vi "ISV Calibration.vi"(7 "queue out":refnum<queue>) -> (1 "Channel Values":dbl[](array[numeric]), 2 "Suceeded":bool, 3 "ADC Table":T1[](array[typedef]))   [LabVIEW 2015]
uses:
  Type/_RT Configuration 2.ctl
  Type/_RT Command.ctl
  Print.ctl
  Configuration/_Global Configuration.vi
  <vilib>/printing/EasyPrintingControls.llb/orientation.ctl
  <vilib>/Utility/NIReport.llb/NI_ReportGenerationCore.lvlib
  <vilib>/printing/EasyPrintingControls.llb/panel_scaling_for_page.ctl
  <vilib>/printing/EasyPrintingControls.llb/margin_values.ctl
  <vilib>/printing/EasyPrintingControls.llb/measurement_system.ctl
  <vilib>/printing/EasyPrintingControls.llb/margins.ctl
  <vilib>/printing/EasyPrintingControls.llb/printing_method.ctl
  <vilib>/printing/EasyPrintingControls.llb/color_or_monochrome.ctl
  <vilib>/printing/EasyPrintingControls.llb/printer_options.ctl
  <vilib>/printing/EasyPrintingControls.llb/page_headers.ctl
  <vilib>/printing/EasyPrintingControls.llb/page_header_content_options.ctl
  <vilib>/printing/EasyPrintingControls.llb/page_header_options.ctl
  <vilib>/printing/EasyPrintingControls.llb/layout_options.ctl
  <vilib>/printing/EasyPrinting.llb/Easy Print VI Panel or Documentation (path).vi
panel:
  out "Progress Bar":u8(slide) scale=0.0..8.0
  out "Error Out":errorcluster
  in  "Error In":errorcluster
  in  "Print":bool
  in  "ADC Channel Calibration":string[][](table)=[["CAP", "104", "0", "", "1000"], ["ISV1", "107", "0", "", "5850"], ["ISV2", "109", "0", "", "5850"]]
  in  "Done":bool
  in  "Start":bool
  out "Current Task":string="Press Start Calibration button to begin or Done button to exit"
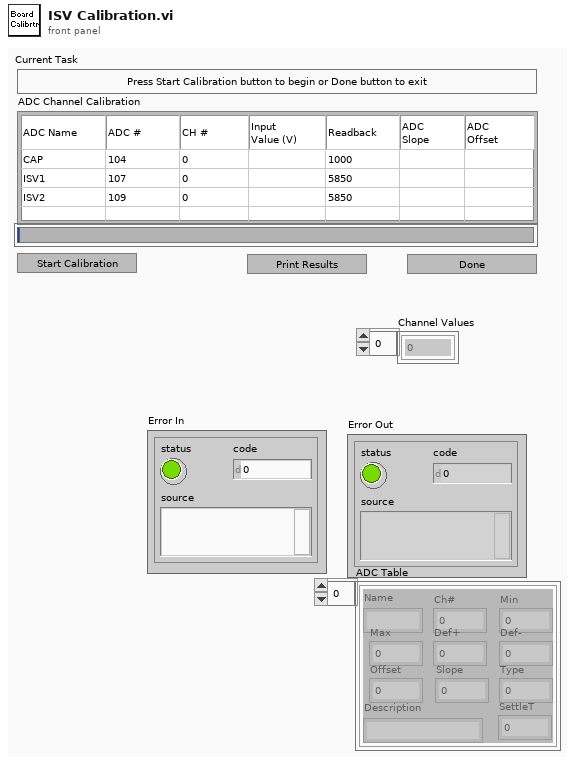
[diagram p1: front panel]
types:
  T1 = typedef "_RT Configuration 2.ctl" = cluster{"Name":string, "Ch#":u8, "Min":dbl, "Max":dbl, "Def+":dbl, "Def-":dbl, "Offset":dbl, "Slope":dbl, "Type":u8, "Description":string, "SettleT":dbl}
  T2 = typedef "_RT Command.ctl" = enum16{"xml Start Run", "xml Start Actual Run", "xml Stop Run", "xml Runtime Update", "xml Get Status", "xml Get Table", "xml Set Table", "xml Get Configuration", "xml System Status", "xml Set LC Input Logic", "xml Get Data", "xml Get Info", "Start", "StartActualRun", "Stop", "Runtime Update", "Get Data", "Get Info", "Get Status", "Get Param", "Get Config", "Get Table", "Read ADC", "Set Oscillator", "Update Config", "Update Table", "Set All Pol", "Set Pol and DC", "Set Max Mass", "Toggle RP", "Toggle EL", "Set PIC", "Initialize Turbo", "Send Turbo Comm", "Close Turbo", "P1", "P2", "P3", "Send Serial", "Set LC Out", "Get LC In", "Read VAC", "Test Table", "Toggle Power", "Get Startup", "Set Startup", "Get ADC Table", "Set ADC Table", "Get Brief Status", "Get Detail Status", "Auxiliary Update", "Set CC Logics", "Set CC Input Logics", "Ignore Error", "invalid"}
  T3 = typedef "Print.ctl" = cluster{"Picture Name":string, "VI Reference":refnum<vi>}
  T4 = typedef "NI_ReportGenerationCore.lvlib/layout_options.ctl" = cluster{"orientation (unchanged)":T5, "panel scaling for page (unchanged)":T6, "margins":T7, "printer options":T10, "page header options":T13}
  T5 = typedef "NI_ReportGenerationCore.lvlib/orientation.ctl" = u16
  T6 = typedef "NI_ReportGenerationCore.lvlib/panel_scaling_for_page.ctl" = u16
  T7 = typedef "NI_ReportGenerationCore.lvlib/margins.ctl" = cluster{"override VI margins (false)":bool, "margins (1.00)":T8, "measurement system (default)":T9}
  T8 = typedef "NI_ReportGenerationCore.lvlib/margin_values.ctl" = cluster{"top":dbl, "left":dbl, "right":dbl, "bottom":dbl}
  T9 = typedef "NI_ReportGenerationCore.lvlib/measurement_system.ctl" = u16
  T10 = typedef "NI_ReportGenerationCore.lvlib/printer_options.ctl" = cluster{"destination printer name (current)":string, "printing method (unchanged)":T11, "color or monochrome (unchanged)":T12}
  T11 = typedef "NI_ReportGenerationCore.lvlib/printing_method.ctl" = u16
  T12 = typedef "NI_ReportGenerationCore.lvlib/color_or_monochrome.ctl" = u16
  T13 = typedef "NI_ReportGenerationCore.lvlib/page_header_options.ctl" = cluster{"page headers (unchanged)":T14, "page header content options":T15}
  T14 = typedef "NI_ReportGenerationCore.lvlib/page_headers.ctl" = u16
  T15 = typedef "NI_ReportGenerationCore.lvlib/page_header_content_options.ctl" = cluster{"Include VI Name":bool, "Include VI Path":bool, "Include Last Modification Date":bool, "Include Date Printed":bool, "Include Page Number":bool, "Include VI Icon":bool}
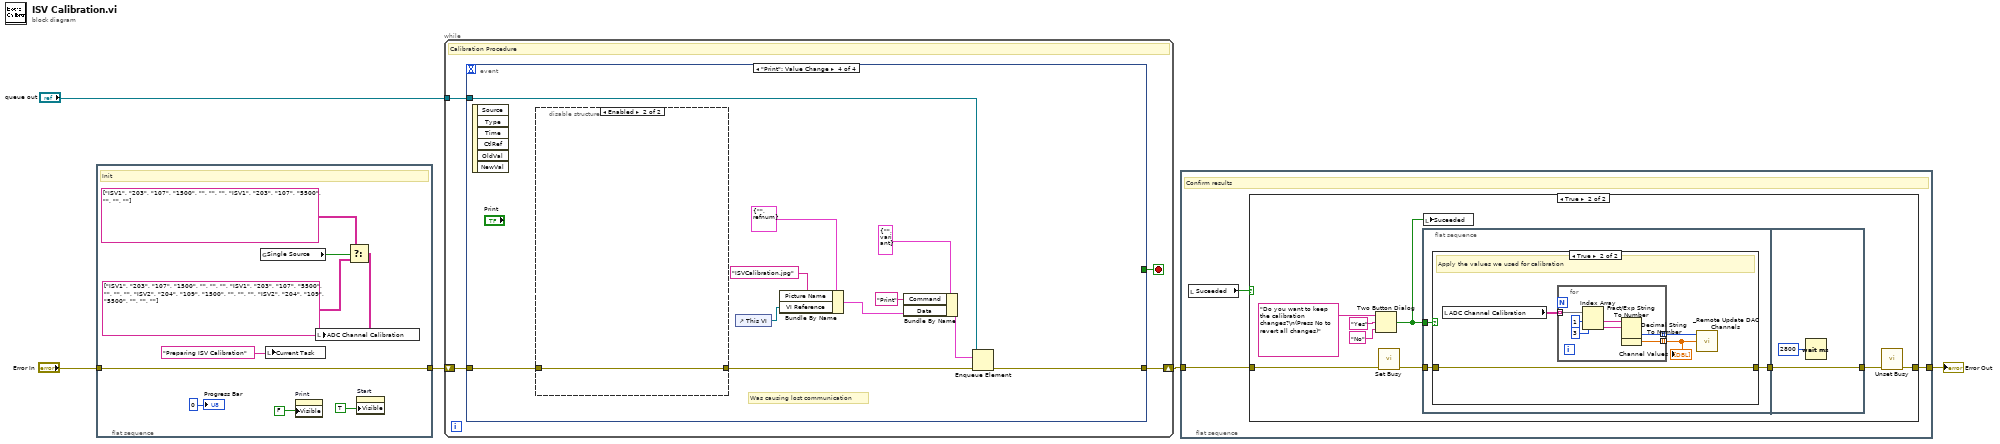
[diagram p0: block diagram]
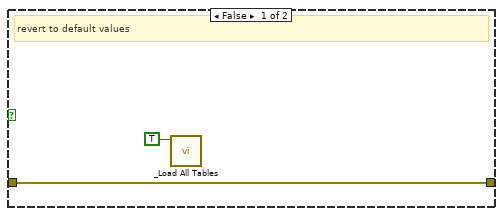
[diagram p3: hidden frame]
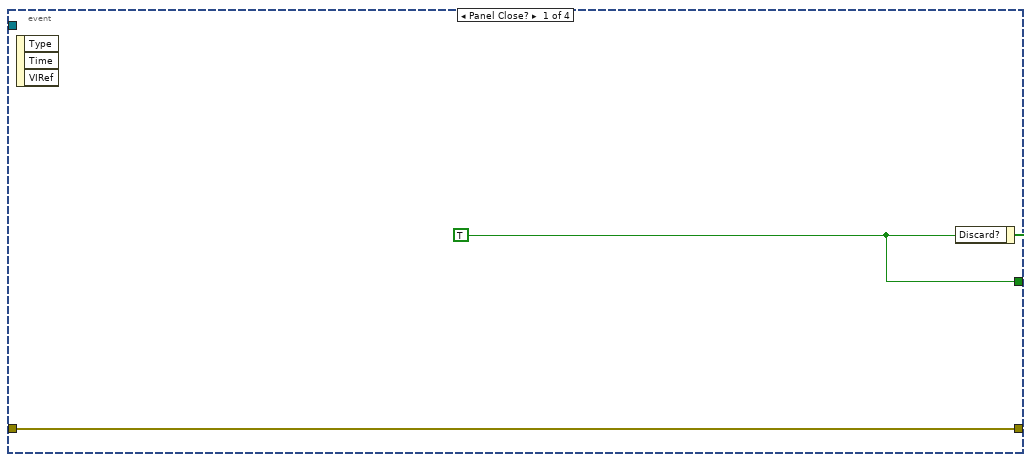
[diagram p4: hidden frame]
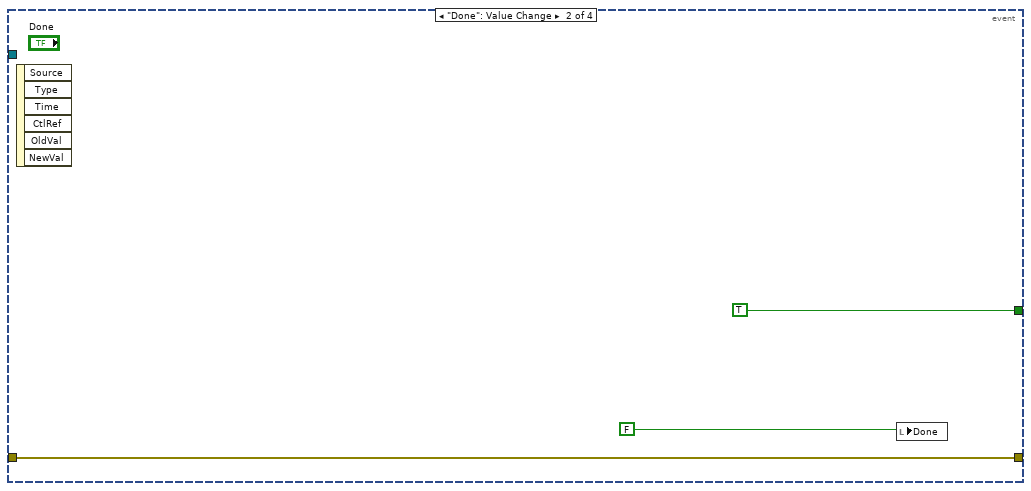
[diagram p5: hidden frame]
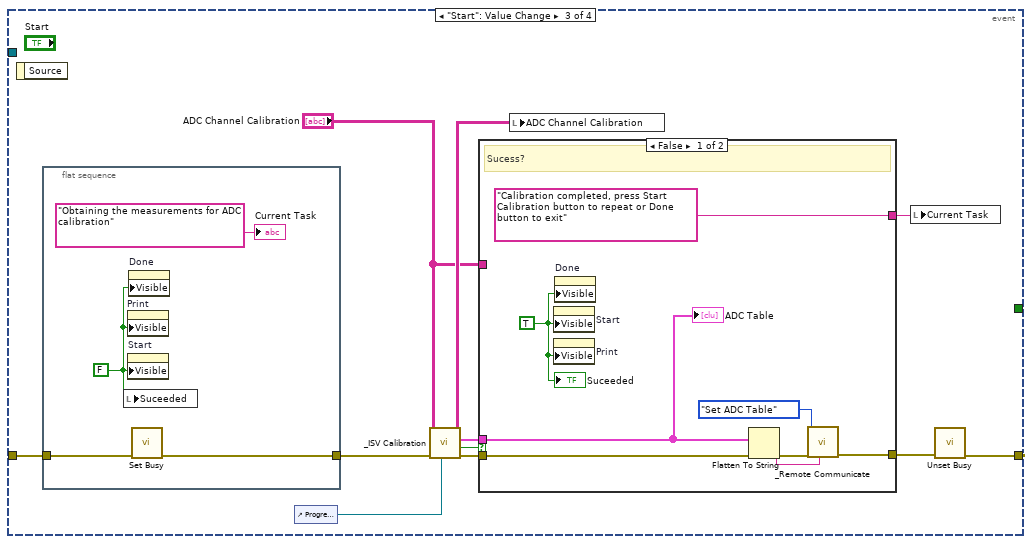
[diagram p6: hidden frame]
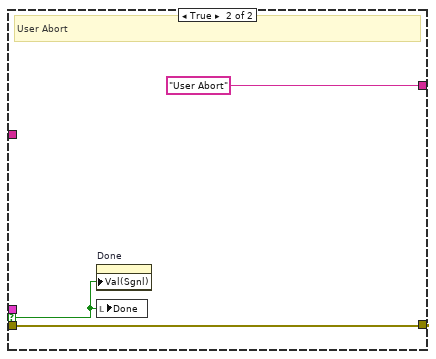
[diagram p7: hidden frame]
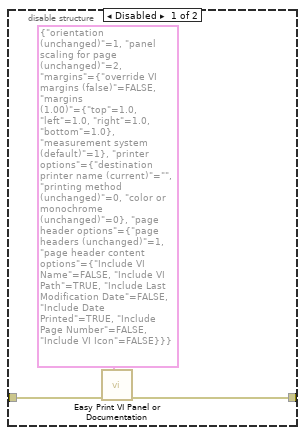
[diagram p8: hidden frame]
diagram:
  n1 = flat-sequence {
    tunnel: "Error In" -> [w11]
    tunnel: [w11] -> w4
    frame #0 {
      # "Init"
      n2 = global read "_Global Configuration.vi" "Single Source"() -> (w10:bool)
      n3 = local write "Current Task"("Preparing ISV Calibration" ("format string")) -> ()
      n4 = property on="Print" class="Bool"("Visible"=FALSE) -> ()  [unwired: 2 in, 2 out]
      n5 = Select(t=string[][] [["ISV1", "203", "107", "1500", "", "", ""], ["ISV1", "203", "107", "5500", "", "", ""]] ("ADC Channel Calibration 2"), s=w10, f=string[][] [["ISV1", "203", "107", "1500", "", "", ""], ["ISV1", "203", "107", "5500", "", "", ""], ["ISV2", "204", "109", "1500", "", "", ""], ["ISV2", "204", "109", "5500", "", "", ""]] ("ADC Channel Calibration 2")) -> (s? t:f=w7:string[][])
      n6 = local write "ADC Channel Calibration"(w7) -> ()
      n7 = property on="Start" class="Bool"("Visible"=TRUE) -> ()  [unwired: 2 in, 2 out]
      "Progress Bar" <- u8 0 ("Progress Bar")
    }
  }
  n8 = while {
    shift-right: [w16] -> w3
    shift-left: w4 -> [w17]
    tunnel: "queue out" -> [w15]
    stop <- w18 stop-if-true
    # "Calibration Procedure"
    n9 = event shown="[3] \"Print\": Value Change" {
      selector: _ -> [_ _ _ _]
      dyn-events: _ -> [_ _ _ _]
      timeout: _ -> [_ _ _ _]
      tunnel: [w20 TRUE _ _] -> w18
      tunnel: w17 -> [w19 w21 w34 w60]
      tunnel: [w19 w21 w33 w58] -> w16
      tunnel: w15 -> [_ _ _ w57]
      event Panel Close? {
        w20 = TRUE
        n10 = event-data() -> ()  [unwired: 4 out]
        n11 = event-data("Discard?"=w20) -> ()  [unwired: 1 in, 1 out]
      }
      event "Done": Value Change {
        n12 = event-data() -> ()  [unwired: 7 out]
        n13 = local write "Done"(FALSE ("Done")) -> ()
      }
      event "Start": Value Change {
        n14 = event-data() -> ()  [unwired: 2 out]
        n15 = flat-sequence {
          tunnel: w34 -> [w38]
          tunnel: [w37] -> w32
          frame #0 {
            w35 = FALSE ("Visible")
            n16 = local write "Suceeded"(w35) -> ()
            n17 = property on="Print" class="Bool"("Visible"=w35) -> ()  [unwired: 2 in, 2 out]
            n18 = property on="Start" class="Bool"("Visible"=w35) -> ()  [unwired: 2 in, 2 out]
            n19 = property on="Done" class="Bool (strict)"("Visible"=w35) -> ()  [unwired: 2 in, 2 out]
            n20 = call <vilib>:"Set Busy.vi"("error in (no error)"=w38) -> ("error out"=w37:errorcluster)  [unwired: 3 in, 7 out]
            "Current Task" <- "Obtaining the measurements for ADC calibration" ("Current Task")
          }
        }
        n21 = control-ref of="Progress Bar"() -> (w24:refnum<vi>)
        n22 = call "_ISV Calibration.vi"("Progress Bar"=w24, "Error In"=w32, "ADC Channel Calibration In"="ADC Channel Calibration") -> ("Error Out"=w31:errorcluster, "aborted"=w30:bool, "ADC Table"=w29:T1[], "ADC Channel Calibration Out"=w26:string[][])  [unwired: 5 in]
        n23 = case shown="False" w30 {
          selector: w30 -> [_ w49]
          tunnel: w31 -> [w45 w48]
          tunnel: w29 -> [w40 _]
          tunnel: [w42 w48] -> w28
          tunnel: ["Calibration completed, press Start Calibration button to repeat or Done button to exit" ("Current Task") "User Abort" ("Current Task")] -> w27
          tunnel: "ADC Channel Calibration" -> [_ _]
          frame False {
            w39 = TRUE ("Visible")
            # "Sucess?"
            n24 = property on="Start" class="Bool"("Visible"=w39) -> ()  [unwired: 2 in, 2 out]
            n25 = property on="Print" class="Bool"("Visible"=w39) -> ()  [unwired: 2 in, 2 out]
            n26 = property on="Done" class="Bool (strict)"("Visible"=w39) -> ()  [unwired: 2 in, 2 out]
            n27 = Flatten To String(anything=w40, error in (no error)=w45) -> (data string=w43:string, error out=w44:errorcluster)  [unwired: 1 in, 2 out]
            n28 = call "_Remote Communicate.vi"("String"=w43, "error in (no error)"=w44, "Command"=_RT_Command."Set ADC Table") -> ("error out"=w42:errorcluster)  [unwired: 3 in, 3 out]
            "Suceeded" <- w39
            "ADC Table" <- w40
          }
          frame True {
            # "User Abort"
            n29 = property on="Done" class="Bool (strict)"("Val(Sgnl)"=w49) -> ()  [unwired: 2 in, 2 out]
            n30 = local write "Done"(w49) -> ()
          }
        }
        n31 = local write "ADC Channel Calibration"(w26) -> ()
        n32 = local write "Current Task"(w27) -> ()
        n33 = call <vilib>:"Unset Busy.vi"("error in (no error)"=w28) -> ("error out"=w33:errorcluster)  [unwired: 1 in, 9 out]
      }
      event "Print": Value Change {
        # "Was causing lost communication"
        n34 = event-data() -> ()  [unwired: 7 out]
        n35 = disable-structure shown="Enabled" {
          disable-tunnel: w60 -> [w62 w64]
          disable-tunnel: [w61 w64] -> w59
          frame Disabled {
            n36 = call-poly <vilib>:"Easy Print VI Panel or Documentation.vi"("layout options"=T4 {"orientation (unchanged)"=1, "panel scaling for page (unchanged)"=2, "margins"={"override VI margins (false)"=FALSE, "margins (1.00)"={"top"=1.0, "left"=1.0, "right"=1.0, "bottom"=1.0}, "measurement system (default)"=1}, "printer options"={"destination printer name (current)"="", "printing method (unchanged)"=0, "color or monochrome (unchanged)"=0}, "page header options"={"page headers (unchanged)"=1, "page header content options"={"Include VI Name"=FALSE, "Include VI Path"=TRUE, "Include Last Modification Date"=FALSE, "Include Date Printed"=TRUE, "Include Page Number"=FALSE, "Include VI Icon"=FALSE}}}, "error in (no error)"=w62) -> ("error out"=w61:errorcluster)  [unwired: 3 in, 6 out]
          }
          frame Enabled {
          }
        }
        n37 = control-ref of="This VI"() -> (w52:refnum<vi>)
        n38 = Bundle By Name(cluster=T3 {"Picture Name"="", "VI Reference"=refnum}, "Picture Name"="ISVCalibration.jpg", "VI Reference"=w52) -> (w51:T3)
        n39 = Bundle By Name(cluster=cluster{"Command":string, "Data":variant} {"Command"="", "Data"=variant} ("element"), "Command"="Print", "Data"=w51) -> (w55:cluster{"Command":string, "Data":variant})
        n40 = Enqueue Element(queue=w57, element=w55, error in (no error)=w59) -> (error out=w58:errorcluster)  [unwired: 1 in, 2 out]
      }
    }
  }
  n41 = flat-sequence {
    tunnel: w3 -> [w65]
    tunnel: [w66] -> w2
    frame #0 {
      # "Confirm results"
      n42 = local read "Suceeded"() -> (w67:bool)
      n43 = case shown="True" w67 {
        tunnel: [w68 w73] -> w66
        tunnel: w65 -> [w68 w74]
        frame False {
        }
        frame True {
          n44 = Two Button Dialog(message="Do you want to keep the calibration changes?\n(Press No to revert all changes)" ("format string"), 1:"No" ("F button name (\"Cancel\")"), 2:"Yes" ("T button name (\"OK\")")) -> (T button?=w69:bool)
          n45 = call <vilib>:"Set Busy.vi"("error in (no error)"=w74) -> ("error out"=w70:errorcluster)  [unwired: 3 in, 7 out]
          n46 = flat-sequence {
            tunnel: [w79] -> w72
            tunnel: w70 -> [w78]
            tunnel: w69 -> [w80]
            tunnel: [w94] -> w71
            tunnel: w72 -> [w94]
            frame #0 {
              n47 = case shown="True" w80 {
                tunnel: [w81 w86] -> w79
                tunnel: w78 -> [w81 w86]
                frame False {
                  # "revert to default values"
                  n48 = call "_Load All Tables.vi"("Use temporary file (F)"=TRUE) -> ()  [unwired: 7 out]
                }
                frame True {
                  # "Apply the values we used for calibration"
                  n49 = local read "ADC Channel Calibration"() -> (w83:string[][])
                  n50 = for {
                    tunnel: w83 -> [w93] mode=indexing
                    tunnel: [w88] -> w84 mode=indexing
                    tunnel: [w87] -> w85 mode=indexing
                    n51 = Index Array(array=w93, index #1=1 ("index"), index #2=3 ("index")) -> (element #1=w90:string, element #2=w89:string)
                    n52 = Decimal String To Number(string=w90) -> (number=w88:i32)  [unwired: 3 out]
                    n53 = Fract/Exp String To Number(string=w89) -> (number=w87:dbl)  [unwired: 4 out]
                  }
                  "Channel Values" <- w85
                  n54 = call "_Remote Update DAC Channels.vi"("UserValue"=w85, "Ch#"=w84) -> ()  [unwired: 1 in, 2 out]
                }
              }
            }
            frame #1 {
              n55 = Wait (ms)(milliseconds to wait=u32 2800) -> ()  [unwired: 1 out]
            }
          }
          n56 = local write "Suceeded"(w69) -> ()
          n57 = call <vilib>:"Unset Busy.vi"("error in (no error)"=w71) -> ("error out"=w73:errorcluster)  [unwired: 1 in, 9 out]
        }
      }
    }
  }
  "Error Out" <- w2
